vi "CRYSplit Wave Data.vi"(9 "sel channel":i32, 10 "nChannels":i32, 11 "wave data in":i32[](array[numeric])) -> (3 "wave data out":i32[](array[numeric]))   [LabVIEW 2013]
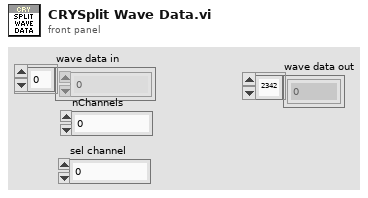
[diagram p1: front panel]
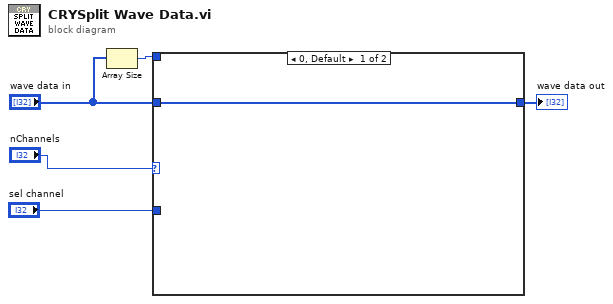
[diagram p0: block diagram]
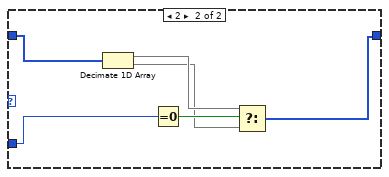
[diagram p2: hidden frame]
diagram:
  n1 = Array Size(array="wave data in") -> (size(s)=w1:i32)
  n2 = case shown="0, Default" "nChannels" {
    tunnel: "wave data in" -> [w6 w12]
    tunnel: [w6 w7] -> w3
    tunnel: "sel channel" -> [_ w10]
    tunnel: w1 -> [_ _]
    frame 0, Default {
    }
    frame 2 {
      n3 = Decimate 1D Array(w12) -> (w9:i32[], w8:i32[])
      n4 = Equal To 0?(x=w10) -> (x = 0?=w11:bool)
      n5 = Select(t=w9, s=w11, f=w8) -> (s? t:f=w7:i32[])
    }
  }
  "wave data out" <- w3
